vi "Write Name.vi"(8 "error in":errorcluster, 10 "Name":string, 11 "Element in":refnum<class "Element.lvclass">) -> (0 "error out":errorcluster, 3 "Element out":refnum<class "Element.lvclass">)   [LabVIEW 2014, in "Element.lvclass"]
uses:
  Element.lvclass
  Element.lvclass/Element.ctl
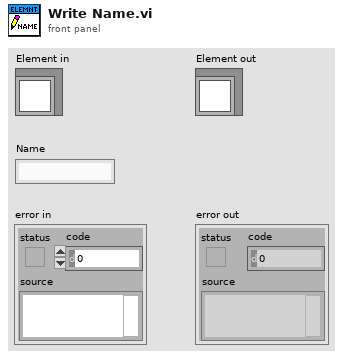
[diagram p1: front panel]
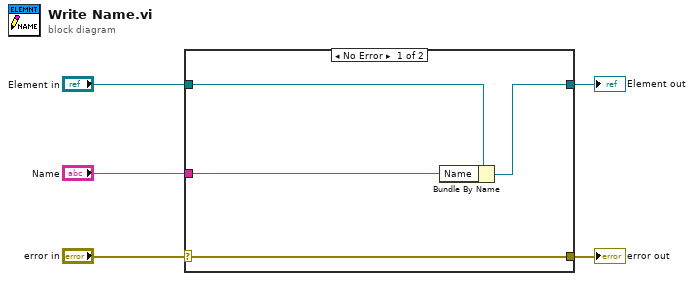
[diagram p0: block diagram]
diagram:
  n1 = case shown="No Error" "error in" {
    selector: "error in" -> [w9 w10]
    tunnel: [w9 w10] -> w4
    tunnel: [w7 w11] -> w2
    tunnel: "Element in" -> [w8 w11]
    tunnel: "Name" -> [w6 _]
    frame No Error {
      n2 = Bundle By Name(cluster=w8, "Name"=w6) -> (w7:refnum<class "Element.lvclass">)
    }
    frame Error {
    }
  }
  "error out" <- w4
  "Element out" <- w2
